vi "Get Info.vi"(8 "error in (no error)":errorcluster, 11 "AChecking in":refnum<class "AChecking.lvclass">) -> (0 "error out":errorcluster, 2 "Account Information":T1, 3 "AChecking out":refnum<class "AChecking.lvclass">)   [LabVIEW 2020, in "AChecking.lvclass"]
uses:
  AChecking.lvclass
  Account Information STYP.ctl
  AChecking.lvclass/AChecking.ctl
  AAccount/AAccount.lvclass
  IInfoable/IInfoable.lvclass
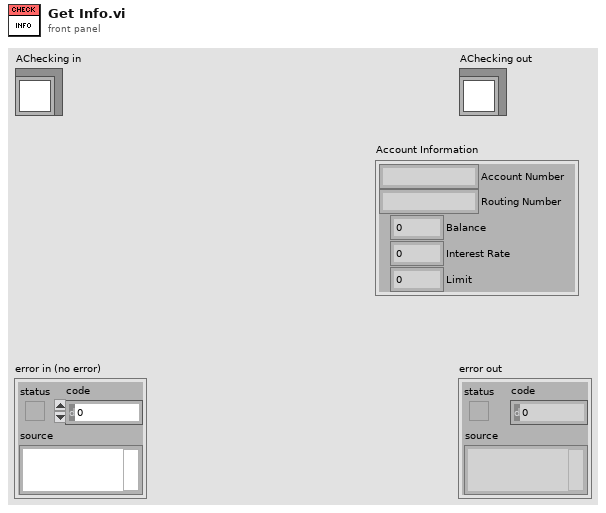
[diagram p1: front panel]
types:
  T1 = typedef "IInfoable.lvclass/Account Information STYP.ctl" = cluster{"Account Number":string, "Routing Number":string, "Balance":dbl, "Interest Rate":dbl, "Limit":dbl}
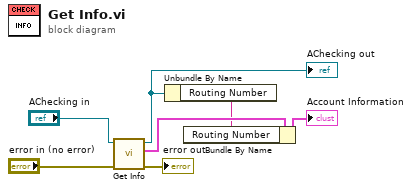
[diagram p0: block diagram]
diagram:
  n1 = call-parent "Get Info.vi"("error in (no error)"="error in (no error)", "AAccount in"="AChecking in") -> ("error out"=→"error out":errorcluster, "Account Information"=w6:T1, "AAccount out"=w2:refnum<class "AChecking.lvclass">)  [unwired: 7 in]
  "AChecking out" <- w2
  n2 = Unbundle By Name(w2) -> ("Routing Number"=w1:string)
  n3 = Bundle By Name(cluster=w6, "Routing Number"=w1) -> (→"Account Information":T1)
